vi "StatisticsGui.FPYcolor.vi"(1 "result":dbl) -> (0 "Color":u32(colorbox))   [LabVIEW 2016]
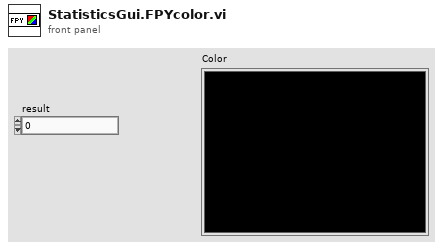
[diagram p1: front panel]
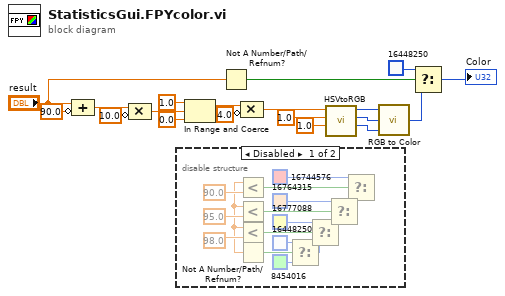
[diagram p0: block diagram]
diagram:
  n1 = Compound Arithmetic op=ADD("result", invert 90.0 ("value")) -> (w1:dbl)
  n2 = Compound Arithmetic op=MULTIPLY(w1, invert 10.0 ("value")) -> (w14:dbl)
  n3 = disable-structure shown="Disabled" {
    frame Disabled {
      n4 = Less?(y=95.0) -> (x=w21:dbl, x < y?=w34:bool)
      n5 = Less?(x=w21, y=90.0) -> (x < y?=w24:bool)
      n6 = Less?(x=w21, y=98.0) -> (x < y?=w31:bool)
      n7 = Not A Number/Path/Refnum?(number/path/refnum=w21) -> (NaN/Path/Refnum?=w28:bool)
      n8 = Select(t=u32 16448250, s=w28, f=u32 8454016) -> (s? t:f=w26:u32)
      n9 = Select(t=u32 16777088, s=w31, f=w26) -> (s? t:f=w30:u32)
      n10 = Select(t=u32 16764315, s=w34, f=w30) -> (s? t:f=w23:u32)
      n11 = Select(t=u32 16744576, s=w24, f=w23) -> ()  [unwired: 1 out]
    }
    frame Enabled {
    }
  }
  n12 = In Range and Coerce(upper limit=1.0, x=w14, lower limit=0.0) -> (coerced(x)=w12:dbl)  [unwired: 1 out]
  n13 = Not A Number/Path/Refnum?(number/path/refnum="result") -> (NaN/Path/Refnum?=w7:bool)
  n14 = Compound Arithmetic op=MULTIPLY(w12, invert 4.0 ("value")) -> (w9:dbl)
  n15 = call "HSVtoRGB.vi"("Value"=1.0 ("Saturation"), "Saturation"=1.0, "Hue [0,1)"=w9) -> ("Blue"=w15:u8, "Green"=w16:u8, "Red"=w17:u8)  [unwired: 6 in]
  n16 = call <vilib>:"RGB to Color.vi"("B"=w15, "G"=w16, "R"=w17) -> ("Color"=w5:u32)
  n17 = Select(t=u32 16448250, s=w7, f=w5) -> (s? t:f=→"Color":u32)
